vi "Parse ipconfig.vi"(8 "error in (no error)":errorcluster, 11 "ipconfig stdout":string) -> (0 "error out":errorcluster, 3 "DNS server addresses":refnum<class "Generic Network Address.lvclass">[](array[class]))   [LabVIEW 2020, in "NI_WFCN.lvlib" / "Hostname Network Address.lvclass"]
doc: "Attempt to locate a configured DNS server."
uses:
  <vilib>/net/WFCN/Addressing/Hostname Network Address/Hostname Network Address.lvclass
  <vilib>/net/WFCN/Addressing/Generic Network Address/Generic Network Address.lvclass
  <vilib>/net/WFCN/Addressing/IPv4 Network Address/IPv4 Network Address.lvclass/IPv4 Network Address.ctl
  <vilib>/net/WFCN/Addressing/Generic Network Address/Generic Network Address.lvclass/Generic Network Address.ctl
  <vilib>/net/WFCN/Addressing/Hostname Network Address/Hostname Network Address.lvclass/Hostname Network Address.ctl
  <vilib>/net/WFCN/Addressing/Hostname Network Address/Create from string.vi
  <vilib>/net/WFCN/Utility/Is IPv4 address.vi
  <vilib>/net/WFCN/Addressing/IPv4 Network Address/Create from U32.vi
  <vilib>/net/WFCN/Addressing/Generic Network Address/Create for unparsable.vi
  <vilib>/net/WFCN/Utility/Is hostname mDNS.vi
  <vilib>/dlg_ctls.llb/Space Constant.vi
  <vilib>/net/WFCN/Addressing/IPv4 Network Address/IPv4 Network Address.lvclass
  e:/builds/penguin/labview/branches/2020/dev/dist/vi.lib/net/WFCN/Addressing/Generic Network Address/Generic Network Address.lvclass
  <vilib>/net/WFCN/Addressing/mDNS Hostname Network Address/mDNS Hostname Network Address.lvclass
  e:/builds/penguin/labview/branches/2020/dev/dist/vi.lib/net/WFCN/Addressing/Hostname Network Address/Hostname Network Address.lvclass
  <vilib>/Utility/error.llb/Error Cluster From Error Code.vi
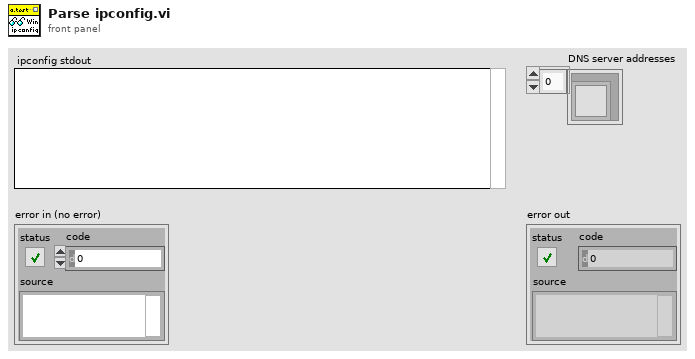
[diagram p1: front panel]
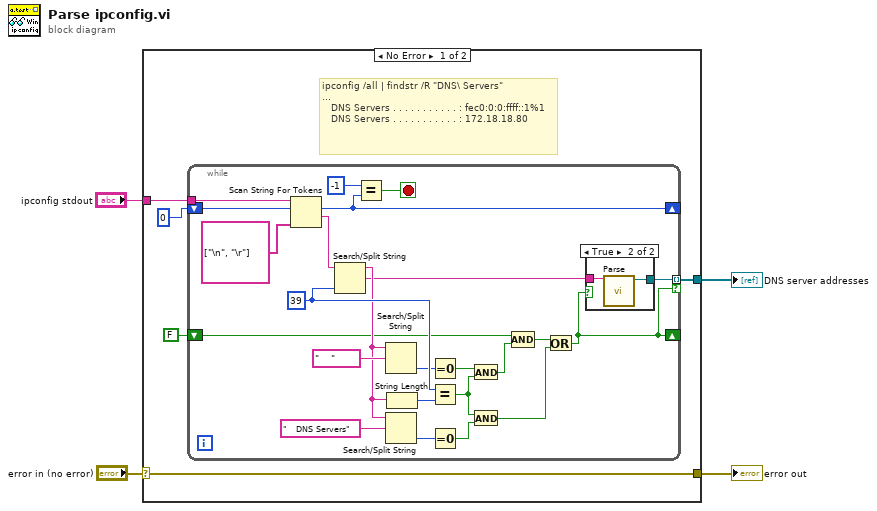
[diagram p0: block diagram]
diagram:
  n1 = case shown="No Error" "error in (no error)" {
    selector: "error in (no error)" -> [w5 w36]
    tunnel: "ipconfig stdout" -> [w7 _]
    tunnel: [w6 _] -> w3
    tunnel: [w5 w36] -> w1
    frame No Error {
      # "ipconfig /all | findstr /R \"DNS\\ Servers\"\n...\n   DNS Servers . . . . . . . . . . . : fec0:0:0:ffff::1%1\n   DNS Servers . . . . . . . . . . . : 172.18.18.80"
      n2 = while {
        shift-right: [w31] -> _
        shift-left: 0 ("offset past token") -> [w32]
        tunnel: w7 -> [w29]
        shift-right: [w10] -> _
        shift-left: FALSE -> [w16]
        tunnel: [w11] -> w6 mode=indexing if=w10
        stop <- w12 stop-if-true
        w25 = 39 ("offset (0)")
        n3 = Scan String For Tokens(6:string[] ["\n", "\r"], 8:w32, 9:w29) -> (1:w28:string, 2:w31:i32)  [unwired: 3 in, 2 out]
        n4 = Search/Split String(string=w28, offset (0)=w25) -> (substring before match=w20:string, match + rest of string=w13:string)  [unwired: 1 in, 1 out]
        n5 = Equal?(x=-1 ("y"), y=w31) -> (x = y?=w12:bool)
        n6 = Search/Split String(string=w20, search string/char (-)="    ") -> (offset of match=w22:i32)  [unwired: 1 in, 2 out]
        n7 = Search/Split String(string=w20, search string/char (-)="   DNS Servers") -> (offset of match=w24:i32)  [unwired: 1 in, 2 out]
        n8 = String Length(string=w20) -> (length=w26:i32)
        n9 = Equal To 0?(x=w22) -> (x = 0?=w19:bool)
        n10 = Equal?(x=w25, y=w26) -> (x = y?=w18:bool)
        n11 = Equal To 0?(x=w24) -> (x = 0?=w23:bool)
        n12 = And(x=w19, y=w18) -> (x .and. y?=w17:bool)
        n13 = And(x=w18, y=w23) -> (x .and. y?=w14:bool)
        n14 = Compound Arithmetic op=AND(w16, w17) -> (w15:bool)
        n15 = Or(x=w15, y=w14) -> (x .or. y?=w10:bool)
        n16 = case shown="True" w10 {
          tunnel: w13 -> [_ w35]
          tunnel: [_ w34] -> w11
          frame False {
          }
          frame True {
            n17 = call <vilib>:"Parse.vi"("address string"=w35) -> ("address"=w34:refnum<class "Generic Network Address.lvclass">)  [unwired: 10 in]
          }
        }
      }
    }
    frame Error {
    }
  }
  "DNS server addresses" <- w3
  "error out" <- w1
